vi "Cause Error.vi"(4 "writer recovery? (T)":bool=TRUE, 6 "formatter recovery? (T)":bool=TRUE, 8 "error in (no error)":errorcluster, 9 "writer error? (F)":bool, 10 "formatter error? (F)":bool, 11 "ini file path":path) -> (0 "error out":errorcluster, 3 "ini file path":path)   [LabVIEW 2018, in "Test Handler.lvclass"]
uses:
  Test Handler.lvclass
  <vilib>/Utility/config.llb/Write Key (Boolean).vi
  <vilib>/Utility/config.llb/NI_LVConfig.lvlib
panel:
  # "Connector Pane"
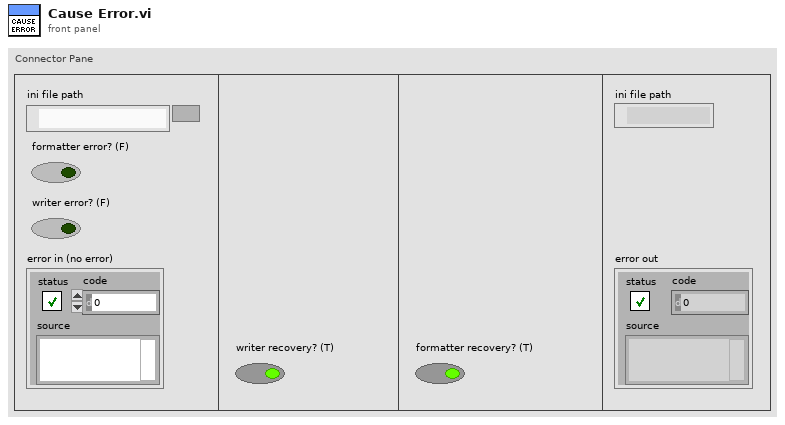
[diagram p1: front panel]
types:
  T1 = typedef "NI_LVConfig.lvlib/Config Data RefNum.ctl" = refnum<k1>
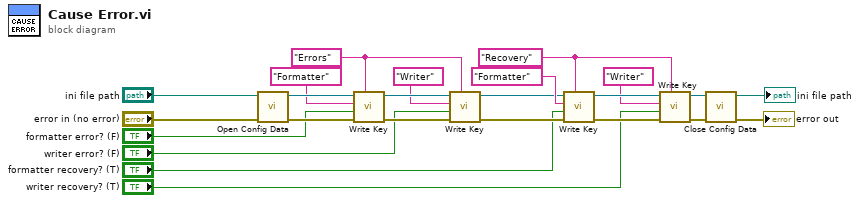
[diagram p0: block diagram]
diagram:
  w8 = "Recovery" ("section")
  w14 = "Errors" ("section")
  n1 = call <vilib>:"Open Config Data.vi"("error in (no error)"="error in (no error)", "configuration file path"="ini file path") -> ("error out"=w18:errorcluster, "refnum"=w21:T1)  [unwired: 7 in, 1 out]
  n2 = call-poly <vilib>:"Write Key.vi"("section"=w14, "error in (no error)"=w18, "value"="formatter error? (F)", "key"="Formatter", "refnum"=w21) -> ("error out"=w23:errorcluster, "refnum out"=w22:T1)  [unwired: 4 in, 1 out]
  n3 = call-poly <vilib>:"Write Key.vi"("section"=w14, "error in (no error)"=w23, "value"="writer error? (F)", "key"="Writer", "refnum"=w22) -> ("error out"=w6:errorcluster, "refnum out"=w4:T1)  [unwired: 4 in, 1 out]
  n4 = call-poly <vilib>:"Write Key.vi"("section"=w8, "error in (no error)"=w6, "value"="formatter recovery? (T)", "key"="Formatter", "refnum"=w4) -> ("error out"=w11:errorcluster, "refnum out"=w10:T1)  [unwired: 4 in, 1 out]
  n5 = call-poly <vilib>:"Write Key.vi"("section"=w8, "error in (no error)"=w11, "value"="writer recovery? (T)", "key"="Writer", "refnum"=w10) -> ("error out"=w5:errorcluster, "refnum out"=w3:T1)  [unwired: 4 in, 1 out]
  n6 = call <vilib>:"Close Config Data.vi"("error in (no error)"=w5, "refnum"=w3) -> ("error out"=→"error out":errorcluster, "file path"=→"ini file path":path)  [unwired: 8 in]
